vi "IstWerte Anzeige.vi"(8 "error in (no error)":errorcluster caption="Fehler (Eingang, kein Fehler)", 11 "Gaskomponete":u16) -> (0 "error out":errorcluster caption="Fehler (Ausgang)", 1 "Standardabweichung":sgl format="%.2f", 2 "Rohwerte":sgl format="%.2f", 3 "Messwerte":sgl format="%.2f")   [LabVIEW 2020, in "Linearisierung v2.lvlib"]
uses:
  Linearisierung v2.lvlib
  Messdaten/Aktionen FGV Messdaten.ctl
  Aktion FGV Rohmesswerte sammeln.ctl
  Seiten/FT-IR/Aktionen EVID-Codes.ctl
  Seiten/FT-IR/FGV FT-IR Aktionen.ctl
  Messdaten/Gewichtung (Stichprobe).ctl
  Messdaten/Messdaten.lvlib
  Seiten/FT-IR/FT-IR.lvlib
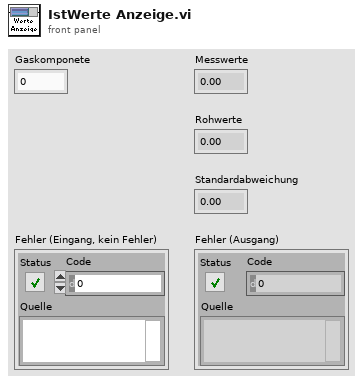
[diagram p1: front panel]
types:
  T1 = typedef "Messdaten.lvlib/Gewichtung (Stichprobe).ctl" = enum16{"Sample", "Population"}
  T2 = typedef "FT-IR.lvlib/FGV FT-IR Aktionen.ctl" = enum16{"lesen", "NOG setzen", "NOS setzen", "Initialisieren", "speichern", "ALLES setzen", "FT-IR Spektrum loggen", "Komm Stoppen", "Spektrum LogKonfig"}
  T3 = typedef "FT-IR.lvlib/Aktionen EVID-Codes.ctl" = enum16{"lesen", "setzen", "laden", "speichern", "1Hz/5Hz", "Smoothing", "Rolling Average"}
  T4 = typedef "Linearisierung v2.lvlib/Aktion FGV Rohmesswerte sammeln.ctl" = enum16{"lesen", "schreiben", "löschen", "Sollwert HovaCal"}
  T5 = typedef "Messdaten.lvlib/Aktionen FGV Messdaten.ctl" = enum16{"lesen", "schreiben", "löschen", "Mittelwerte", "Komponente"}
  T6 = typedef "FT-IR.lvlib/1Hz-5Hz Geraet.ctl" = u16
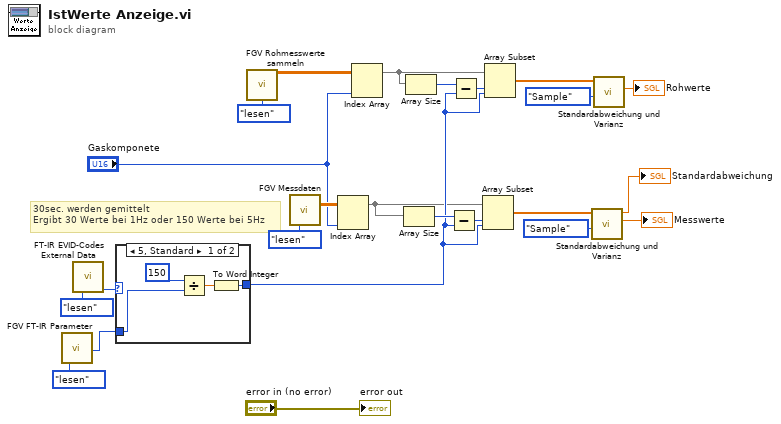
[diagram p0: block diagram]
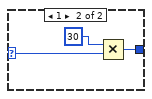
[diagram p2: hidden frame]
diagram:
  # "30sec. werden gemittelt\nErgibt 30 Werte bei 1Hz oder 150 Werte bei 5Hz"
  n1 = call "FGV FT-IR Parameter.vi"("Aktion"=FGV_FT-IR_Aktionen."lesen") -> ("NoOfScan"=w18:u32)  [unwired: 11 in, 7 out]
  n2 = call "FT-IR EVID-Codes External Data.vi"("Aktionen"=Aktionen_EVID-Codes."lesen") -> ("1Hz/5Hz Gerät"=w19:T6)  [unwired: 9 in, 5 out]
  n3 = case shown="5, Standard" w19 {
    selector: w19 -> [_ w29]
    tunnel: [w25 w30] -> w8
    tunnel: w18 -> [w27 _]
    frame 5, Default {
      n4 = Divide(x=150, y=w27) -> (x/y=w26:dbl)
      n5 = To Word Integer(number=w26) -> (16bit integer=w25:i16)
    }
    frame 1 {
      n6 = Multiply(x=30, y=w29) -> (x*y=w30:i32)
    }
  }
  n7 = call "FGV Rohmesswerte sammeln.vi"("Aktion"=Aktion_FGV_Rohmesswerte_sammeln."lesen") -> ("Rohmessdaten"=w17:sgl[][])  [unwired: 11 in, 3 out]
  n8 = call "FGV Messdaten.vi"("Aktionen"=Aktionen_FGV_Messdaten."lesen") -> ("Messdaten"=w23:sgl[][])  [unwired: 6 in, 8 out]
  n9 = Index Array(array=w23, index (col)="Gaskomponete") -> (element=w6:sgl[])  [unwired: 1 in]
  n10 = Index Array(array=w17, index (col)="Gaskomponete") -> (element=w7:sgl[])  [unwired: 1 in]
  n11 = Array Size(array=w6) -> (size(s)=w16:i32)
  n12 = Array Size(array=w7) -> (size(s)=w9:i32)
  n13 = Subtract(x=w16, y=w8) -> (x-y=w15:i32)
  n14 = Subtract(x=w9, y=w8) -> (x-y=w10:i32)
  n15 = Array Subset(array=w6, index=w15, length=w8) -> (w13:sgl[])
  n16 = Array Subset(array=w7, index=w10, length=w8) -> (w12:sgl[])
  n17 = call "Standardabweichung und Varianz.vi"("Gewichtung (Stichprobe)"=Gewichtung_(Stichprobe)."Sample", "X"=w13) -> ("Mittelwert"=→"Messwerte":sgl, "Standardabweichung"=→"Standardabweichung":sgl)  [unwired: 7 in, 1 out]
  n18 = call "Standardabweichung und Varianz.vi"("Gewichtung (Stichprobe)"=Gewichtung_(Stichprobe)."Sample", "X"=w12) -> ("Mittelwert"=→"Rohwerte":sgl)  [unwired: 7 in, 2 out]
  "error out" <- "error in (no error)"
